vi "publishILCInputs.vi"(8 "error in (no error)":errorcluster, 11 "Model in":refnum<class "Model.lvclass">) -> (0 "error out":errorcluster, 3 "Model out":refnum<class "Model.lvclass">)   [LabVIEW 2015, in "Model.lvclass"]
uses:
  Model.lvclass
  Typedefs/ADC Outputs.ctl
  Model.lvclass/Model.ctl
  <userlib>/Common/ILC/ILC/ILC.lvclass/ILC.ctl
  UserEvents/UserEvents.lvclass/UserEvents.ctl
  UserEvents/UserEvents.lvclass
  <userlib>/Common/ILC/ILC/ILC.lvclass
  Typedefs/FAMTTypedefs.lvlib
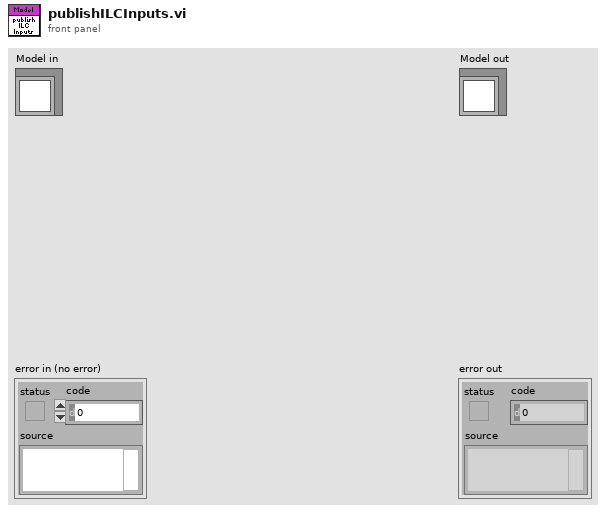
[diagram p1: front panel]
types:
  T1 = typedef "FAMTTypedefs.lvlib/ADC Outputs.ctl" = cluster{"Ch1":dbl[unit], "Ch2":dbl[unit], "Ch3":dbl[unit], "Ch4":dbl[unit]}
  T2 = typedef "ILCCommon.lvlib/ILCTypedefs.lvlib/ADC Eng.ctl" = cluster{"Ch1":dbl[unit], "Ch2":dbl[unit], "Ch3":dbl[unit], "Ch4":dbl[unit]}
  T3 = typedef "FAMTTypedefs.lvlib/PubDataEvents.ctl" = cluster{"State":refnum<user-event>, "ErrorCode":refnum<user-event>, "ADC Outputs":refnum<user-event>, "InputData":refnum<user-event>, "ControllerData":refnum<user-event>, "TestStatus":refnum<user-event>, "LogPath":refnum<user-event>}
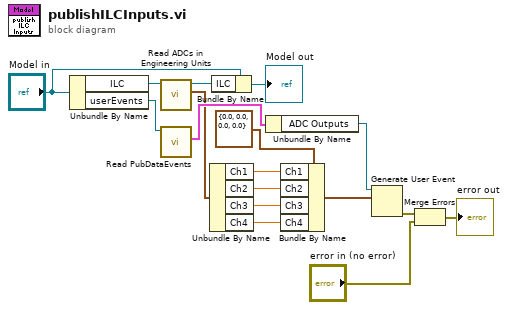
[diagram p0: block diagram]
diagram:
  n1 = Unbundle By Name("Model in") -> ("ILC"=w15:refnum<class "ILC.lvclass">, "userEvents"=w17:refnum<class "UserEvents.lvclass">)
  n2 = call <userlib>:"Read ADCs in Engineering Units.vi"("ILC in"=w15) -> ("ADCs in Engineering Units"=w13:T2, "ILC out"=w3:refnum<class "ILC.lvclass">)  [unwired: 9 in]
  n3 = call "Read PubDataEvents.vi"("UserEvents in"=w17) -> ("PubDataEvents"=w16:T3)  [unwired: 9 in, 1 out]
  n4 = Unbundle By Name(w13) -> ("Ch1"=w1:dbl[unit], "Ch2"=w12:dbl[unit], "Ch3"=w11:dbl[unit], "Ch4"=w10:dbl[unit])
  n5 = Bundle By Name(cluster="Model in", "ILC"=w3) -> (→"Model out":refnum<class "Model.lvclass">)
  n6 = Unbundle By Name(w16) -> ("ADC Outputs"=w9:refnum<user-event>)
  n7 = Bundle By Name(cluster=T1 {"Ch1"=0.0, "Ch2"=0.0, "Ch3"=0.0, "Ch4"=0.0} ("Output Data"), "Ch1"=w1, "Ch2"=w12, "Ch3"=w11, "Ch4"=w10) -> (w8:T1)
  n8 = Generate User Event(user event=w9, event data cluster=w8) -> (error out=w7:errorcluster)  [unwired: 2 in, 1 out]
  n9 = Merge Errors(w7, "error in (no error)") -> (→"error out":errorcluster)
